vi "re_DataLog Tag Info.vi"(0 "database ref (use name)":T7, 1 "flush? (false)":bool, 5 "database (current)":string, 7 "tag":string, 9 "tag index (use tag)":i32=-1, 11 "error in (no error)":errorcluster) -> (4 "tag log directory":path, 6 "tag config":T1 {"logging parameters" format="%.2e"; "precision" items=["0", "1", "2", "3", "4", "5", "6", "7", "8", "9", "10", "11", "12", "13", "14", "15", "16", "17"]; "limit delay" format="%.2e"; "deadband" format="%.2e"}, 8 "mode":T6, 15 "error out":errorcluster)   [LabVIEW 2012]
doc: "Return information on a tag in a database. The returned tag log directory can be used to perform queries on the tag's log. The returned tag config cluster can be used to determin the temporal type, value type, or unit of the tag.\n\nThe tag can be specified via its name, or via its index. In the latter case the database must be live. The database can be specified via a reference or name. When omitting both, the current database is used.\n\nWhen true is wired to the flush input, an attempt will be made to flush the buffered tag data to the log before returning. Use this when you are about to query data from the log and require the most recent available data. Note that flushing propagates over the network for a mirrored database provided that a mirroring connection has been established.\n\nThis VI is reentrant not only because flushing might take some time, but also to avoid recursion deadlocks when the database being mirrored is part of the local runtime (e.g. for testing purposes)."
uses:
  typedefs/t_DataLog Database Info Pane.ctl
  typedefs/clusters/t_DataLog Tag Config.ctl
  typedefs/t_DataLog Temporal Types.ctl
  typedefs/t_DataLog Value Types.ctl
  typedefs/t_DataLog Numerical Format.ctl
  typedefs/t_DataLog Logging Algorithms.ctl
  typedefs/t_Datalog Datebase Modes.ctl
  typedefs/t_DataLog Tag Info List Methods.ctl
  typedefs/t_DataLog Databases Methods.ctl
  typedefs/t_DataLog Tag Hash Methods.ctl
  typedefs/t_DataLog Aggregate New Points Methods.ctl
  typedefs/t_DataLog Aggregation Buffer Methods.ctl
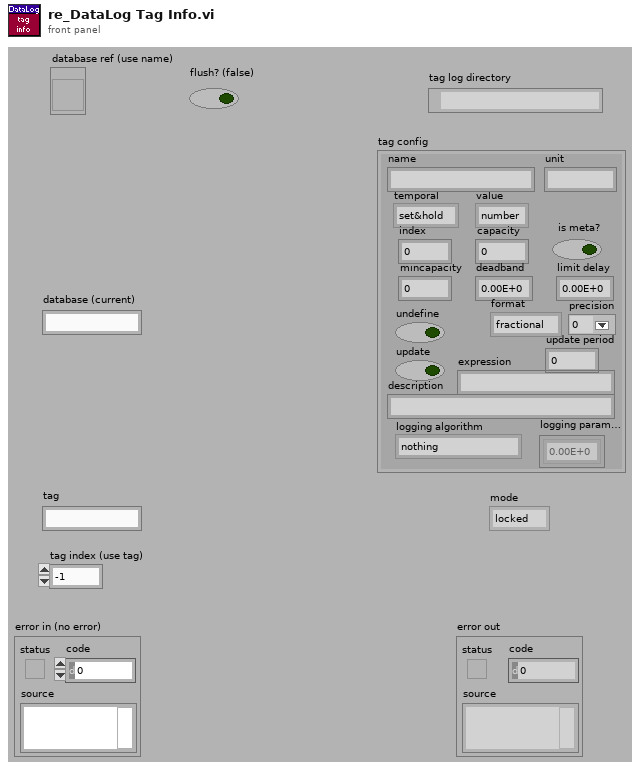
[diagram p1: front panel]
types:
  T1 = typedef "t_DataLog Tag Config.ctl" = cluster{"name":string, "unit":string, "temporal":T2, "value":T3, "index":i32, "capacity":i32, "is meta?":bool, "mincapacity":i32, "deadband":dbl, "limit delay":dbl, "format":T4, "precision":u8, "undefine":bool, "update":bool, "update period":u16, "expression":string, "description":string, "logging algorithm":T5, "logging parameters":dbl[]}
  T2 = typedef "t_DataLog Temporal Types.ctl" = enum16{"set&hold", "sample", "event"}
  T3 = typedef "t_DataLog Value Types.ctl" = enum16{"number", "string"}
  T4 = typedef "t_DataLog Numerical Format.ctl" = enum8{"fractional", "exponential", "engineering"}
  T5 = typedef "t_DataLog Logging Algorithms.ctl" = enum16{"nothing", "changes", "everything", "every Nth", "time threshold", "value threshold + prior", "t or v threshold", "t or v threshold + prior"}
  T6 = typedef "t_Datalog Datebase Modes.ctl" = enum16{"locked", "unlocked", "live", "mirrored"}
  T7 = typedef "t_DataLog Database Info Pane.ctl" = refnum<vi>
  T8 = typedef "t_DataLog Tag Info List Methods.ctl" = enum16{"initialize", "create", "create empty", "rename", "delete", "test tag", "get", "get by name", "get default", "get list", "get path", "get subsets", "set subsets", "set config", "set capacity", "#tags", "go live", "set unlocked", "set mirrored"}
  T9 = typedef "t_DataLog Aggregation Buffer Methods.ctl" = enum16{"initialize", "write", "write special", "flush", "flush next", "flush next if", "setup recovery", "update recovery", "verify recovery", "dummy flush ", "cleanup"}
  T10 = typedef "t_DataLog Aggregate New Points Methods.ctl" = enum16{"initialize", "aggregate", "cleanup"}
  T11 = typedef "t_DataLog Tag Hash Methods.ctl" = enum16{"initialize", "add tag", "index tag", "lookup", "#tags", "cleanup", "write recovery", "read recovery", "delete recovery"}
  T12 = typedef "t_DataLog Databases Methods.ctl" = enum16{"initialize", "get ref", "get names", "cleanup"}
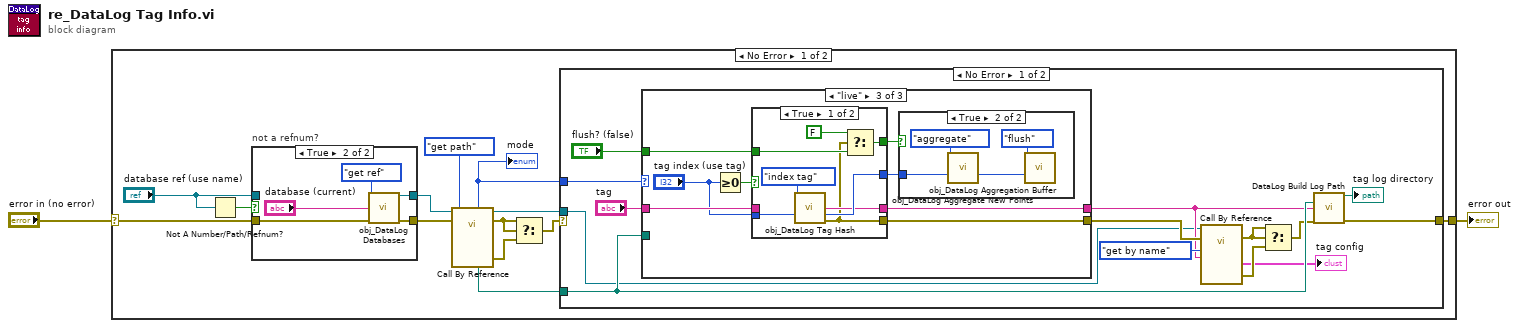
[diagram p0: block diagram]
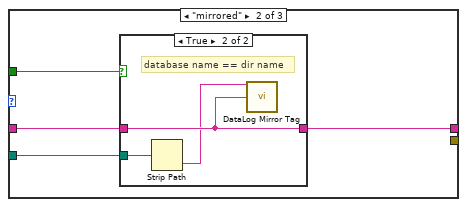
[diagram p3: hidden frame]
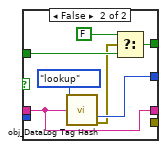
[diagram p6: hidden frame]
diagram:
  n1 = case shown="No Error" "error in (no error)" {
    selector: "error in (no error)" -> [w11 w74]
    tunnel: [w15 w74] -> w2
    frame No Error {
      n2 = Not A Number/Path/Refnum?(number/path/refnum="database ref (use name)") -> (NaN/Path/Refnum?=w7:bool)
      n3 = case "not a refnum?" shown="True" w7 {
        tunnel: [w68 w72] -> w14
        tunnel: w11 -> [w67 w71]
        tunnel: [w67 w70] -> w10
        tunnel: "database ref (use name)" -> [w68 _]
        frame False {
        }
        frame True {
          n4 = call "obj_DataLog Databases.vi"("method"=t_DataLog_Databases_Methods."get ref", "database (current)"="database (current)", "error in (no error)"=w71) -> ("database ref"=w72:T7, "error out"=w70:errorcluster)  [unwired: 10 in, 1 out]
        }
      }
      n5 = call-by-ref "?"(reference=w14, error in=w10, "method"=t_DataLog_Tag_Info_List_Methods."get path") -> (reference out=w3:T7, error out=w9:errorcluster, "mode"=w4:T6, "path"=w12:path, 15:"error out"=w8:errorcluster)  [unwired: 8 in, 4 out]
      "mode" <- w4
      n6 = Select(t=w9, s=w9, f=w8) -> (s? t:f=w5:errorcluster)
      n7 = case shown="No Error" w5 {
        selector: w5 -> [_ w66]
        tunnel: [w28 w66] -> w15
        tunnel: w12 -> [w24 _]
        tunnel: w4 -> [w27 _]
        tunnel: w3 -> [w16 _]
        frame No Error {
          n8 = case shown="\"live\"" w27 {
            tunnel: [_ _ w46] -> w21
            tunnel: [w30 w33 w45] -> w17
            tunnel: "tag" -> [w30 w34 w44]
            tunnel: "flush? (false)" -> [_ w32 w41]
            tunnel: w24 -> [_ w31 _]
            frame "locked", "unlocked" {
            }
            frame "mirrored" {
              n9 = case shown="True" w32 {
                tunnel: w34 -> [w35 w38]
                tunnel: [w35 w38] -> w33
                tunnel: w31 -> [_ w37]
                frame False {
                }
                frame True {
                  # "database name == dir name"
                  n10 = Strip Path(path=w37) -> (name=w36:string)  [unwired: 1 out]
                  n11 = call "DataLog Mirror Tag.vi"("local db"=w36, "tag"=w38) -> ()  [unwired: 12 in, 2 out]
                }
              }
            }
            frame "live" {
              n12 = Greater Or Equal To 0?(x="tag index (use tag)") -> (x >= 0?=w43:bool)
              n13 = case shown="True" w43 {
                tunnel: [w53 _] -> w46
                tunnel: [w56 w64] -> w39
                tunnel: "tag index (use tag)" -> [w57 _]
                tunnel: [w55 w63] -> w45
                tunnel: w44 -> [_ w63]
                tunnel: w41 -> [w54 w62]
                tunnel: [w51 w59] -> w40
                frame True {
                  n14 = call "obj_DataLog Tag Hash.vi"("method"=t_DataLog_Tag_Hash_Methods."index tag", "tag index in"=w57) -> ("tag out"=w55:string, "tag index out"=w56:i32, "error out"=w53:errorcluster)  [unwired: 10 in, 1 out]
                  n15 = Select(t=FALSE, s=w53, f=w54) -> (s? t:f=w51:bool)
                }
                frame False {
                  n16 = call "obj_DataLog Tag Hash.vi"("method"=t_DataLog_Tag_Hash_Methods."lookup", "tag in"=w63) -> ("tag index out"=w64:i32, "error out"=w61:errorcluster)  [unwired: 10 in, 2 out]
                  n17 = Select(t=FALSE, s=w61, f=w62) -> (s? t:f=w59:bool)
                }
              }
              n18 = case shown="True" w40 {
                tunnel: w39 -> [_ w50]
                frame False {
                }
                frame True {
                  n19 = call "obj_DataLog Aggregate New Points.vi"("method"=t_DataLog_Aggregate_New_Points_Methods."aggregate", "tag index in"=w50) -> ("tag index out"=w48:i32)  [unwired: 13 in]
                  n20 = call "obj_DataLog Aggregation Buffer.vi"("method"=t_DataLog_Aggregation_Buffer_Methods."flush", "tag index"=w48) -> ()  [unwired: 12 in, 2 out]
                }
              }
            }
          }
          n21 = call-by-ref "?"(reference=w16, error in=w21, "method"=t_DataLog_Tag_Info_List_Methods."get by name", "tag or base tag"=w17) -> (error out=w23:errorcluster, "tag config out"=→"tag config":T1, 15:"error out"=w22:errorcluster)  [unwired: 7 in, 6 out]
          n22 = Select(t=w23, s=w23, f=w22) -> (s? t:f=w20:errorcluster)
          n23 = call "DataLog Build Log Path.vi"("database path"=w24, "tag"=w17, "error in (no error)"=w20) -> ("tag log directory"=→"tag log directory":path, "error out"=w28:errorcluster)  [unwired: 11 in]
        }
        frame Error {
        }
      }
    }
    frame Error {
    }
  }
  "error out" <- w2
